vi "写入V4版外设配置.vi"(8 "error in (no error)":errorcluster, 10 "外设配置":T1 {"阀型号" items=["垦拓10通阀"]; "总氮x公式0" items=["0", "1"]; "光谱仪类型" items=["1型", "2型", "3型", "2型氙灯联控"]; "泵类型" items=["润泽注射泵", "垦拓注射泵"]}, 11 "MB session in":refnum<class "MB_Master.lvclass">) -> (0 "error out":errorcluster, 3 "MB session out":refnum<class "MB_Master.lvclass">)   [LabVIEW 2022 SP3, in "斯坦道总氮.lvlib"]
uses:
  <vilib>/Plasmionique/MB Master/MB_Master/MB_Master.lvclass
  <vilib>/Plasmionique/MB Master/MB_Master_Serial/MB_Master_Serial.lvclass
  C:/Program Files (x86)/National Instruments/LabVIEW 2022/vi.lib/Plasmionique/MB Master/MB_Master/MB_Master.lvclass
  <vilib>/Plasmionique/MB Master/MB Master.lvlib
panel:
  out "大小":i32
  in  "U32":u32
  in  "SGL":sgl
  in  "U16":u16
  in  "U8":u8
  in  "VISA Resource":refnum<visa-resource-name>
  in  "引用选择":enum16{"MB引用", "自建引用"}(ring)
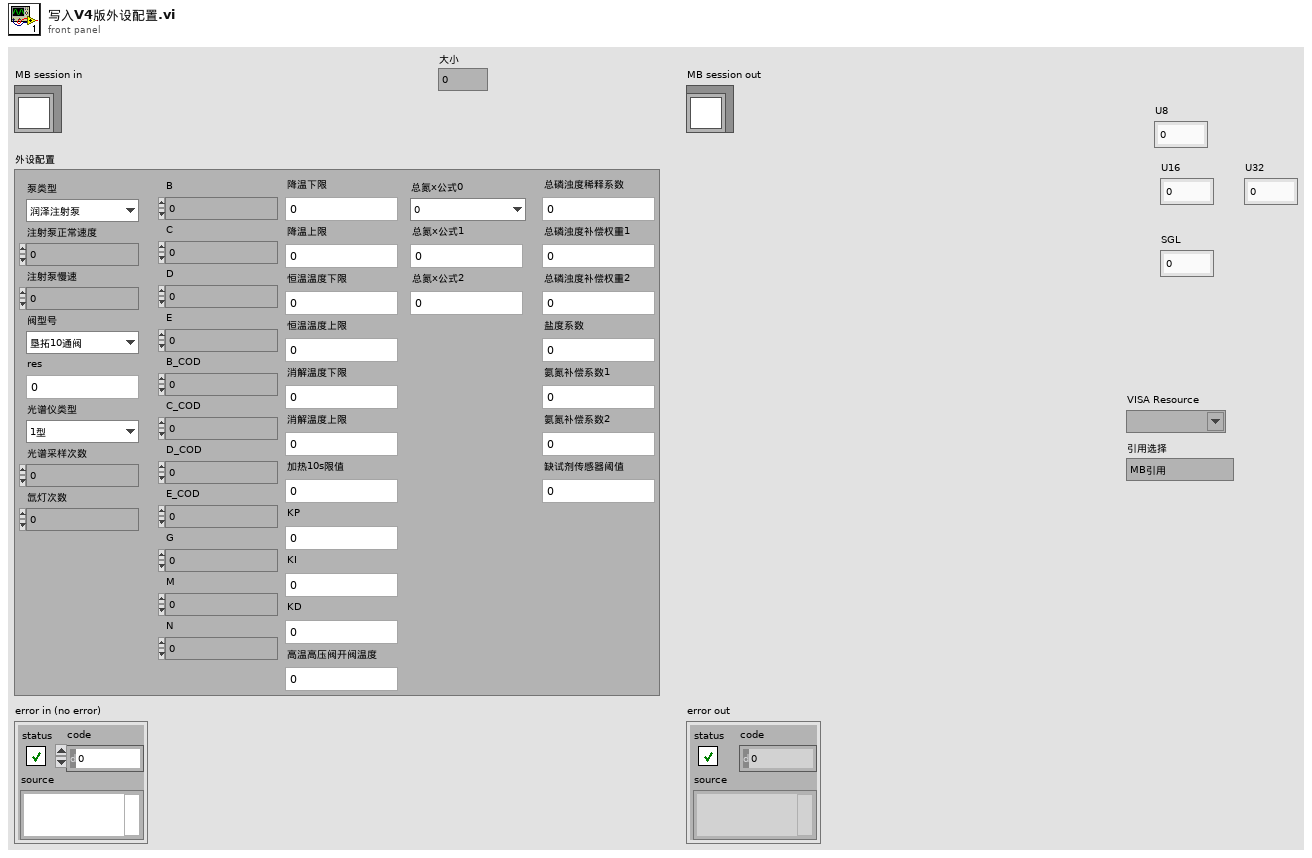
[diagram p1: front panel]
types:
  T1 = typedef "斯坦道总氮.lvlib/V4版外设参数.ctl" = cluster{"泵类型":u8, "注射泵正常速度":u32, "注射泵慢速":u32, "阀型号":u8, "res":u8, "光谱仪类型":u8, "光谱采样次数":u8, "氙灯次数":u8, "B":u16, "C":u16, "D":u16, "E":u16, "B_COD":u16, "C_COD":u16, "D_COD":u16, "E_COD":u16, "G":u16, "M":u16, "N":u16, "降温下限":sgl, "降温上限":sgl, "恒温温度下限":sgl, "恒温温度上限":sgl, "消解温度下限":sgl, "消解温度上限":sgl, "加热10s限值":sgl, "KP":sgl, "KI":sgl, "KD":sgl, "高温高压阀开阀温度":sgl, "总氮x公式0":u8, "总氮x公式1":sgl, "总氮x公式2":sgl, "总磷浊度稀释系数":sgl, "总磷浊度补偿权重1":sgl, "总磷浊度补偿权重2":sgl, "盐度系数":sgl, "氨氮补偿系数1":sgl, "氨氮补偿系数2":sgl, "缺试剂传感器阈值":u16}
  T2 = cluster{"baud rate (bps)":u32, "stop bits":u16, "parity":u16, "flow control":u16, "timeout":u32, "retries":i32}
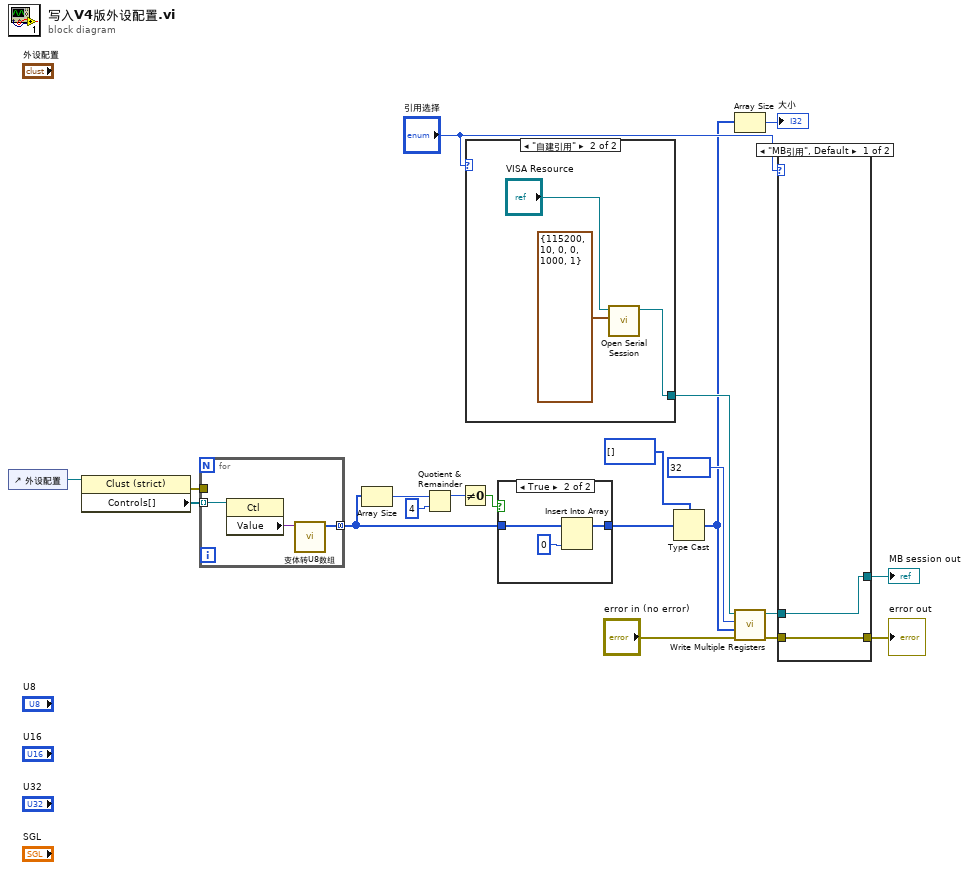
[diagram p0: block diagram]
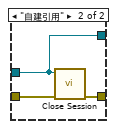
[diagram p3: hidden frame]
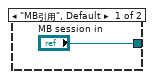
[diagram p4: hidden frame]
diagram:
  n1 = control-ref of="外设配置"() -> (w10:refnum<vi>)
  n2 = property class="Clust (strict)"(reference=w10) -> (error out=w1:errorcluster, "Controls[]"=w12:refnum<vi>[])  [unwired: 1 in, 1 out]
  n3 = for {
    tunnel: w12 -> [w23] mode=indexing
    tunnel: [w21] -> w3 mode=concatenating
    tunnel: w1 -> [_]
    n4 = property class="Ctl"(reference=w23) -> ("Value"=w22:variant)  [unwired: 1 in, 2 out]
    n5 = call "变体转U8数组.vi"("Value"=w22) -> ("U8数组"=w21:u8[])  [unwired: 9 in, 1 out]
  }
  n6 = Array Size(array=w3) -> (size(s)=w6:i32)
  n7 = Quotient & Remainder(x=w6, y=4) -> (x-y*floor(x/y)=w5:i32)  [unwired: 1 out]
  n8 = Not Equal To 0?(x=w5) -> (x != 0?=w4:bool)
  n9 = case shown="\"自建引用\"" "引用选择" {
    tunnel: ["MB session in" w27] -> w18
    frame "MB引用", Default {
    }
    frame "自建引用" {
      n10 = call <vilib>:"Open Serial Session.vi"("Serial Config"=T2 {"baud rate (bps)"=115200, "stop bits"=10, "parity"=0, "flow control"=0, "timeout"=1000, "retries"=1}, "VISA Resource"="VISA Resource") -> ("MB_Serial session"=w27:refnum<class "MB_Master_Serial.lvclass">)  [unwired: 8 in, 1 out]
    }
  }
  n11 = case shown="True" w4 {
    tunnel: w3 -> [w28 w31]
    tunnel: [w28 w29] -> w2
    frame False {
    }
    frame True {
      n12 = Insert Into Array(array=w31, new element=u8 0 ("新元素/子数组")) -> (w29:u8[])  [unwired: 1 in]
    }
  }
  n13 = Type Cast(type=u16[] [], x=w2) -> (*(type *) &x=w9:u16[])
  n14 = Array Size(array=w9) -> (size(s)=→"大小":i32)
  n15 = call <vilib>:"Write Multiple Registers.vi"("error in (no error)"="error in (no error)", "values"=w9, "starting address"=u16 32, "MB session in"=w18) -> ("error out"=w15:errorcluster, "MB session out"=w17:refnum<class "MB_Master.lvclass">)  [unwired: 6 in]
  n16 = case shown="\"MB引用\", Default" "引用选择" {
    tunnel: w17 -> [w32 w34]
    tunnel: w15 -> [w33 w36]
    tunnel: [w33 w35] -> w14
    tunnel: [w32 w34] -> w13
    frame "MB引用", Default {
    }
    frame "自建引用" {
      n17 = call-dynamic "Close Session.vi"("error in (no error)"=w36, "MB session in"=w34) -> ("error out"=w35:errorcluster)  [unwired: 9 in]
    }
  }
  "MB session out" <- w13
  "error out" <- w14
